vi "Stepper_motor_control_labview_version_2.0.vi"() -> ()   [LabVIEW 2019]
uses:
  <vilib>/Analysis/baseanly.llb/Mean (DBL).vi
  <vilib>/Waveform/WDTOps.llb/WDT Append Waveforms DBL.vi
  <vilib>/Analysis/NI_AALBase.lvlib
panel:
  out "Distance in cm":dbl
  in  "Stop Sensor CCW":bool
  out "Waveform Chart":waveform(dbl)(graph)
  in  "Stop sensor CW":bool
  in  "CW":bool
  out "DO CW":bool[](array[boolean])
  in  "How many laps CW":i32
  in  "How many laps CCW":i32
  in  "CCW":bool
  out "DO CCW":bool[](array[boolean])
  # "4 Steg = 1,8 x 4 = 7,2\n=> 45/7,2 = 6,25 = 25 varv\n=> 90/7,2 = 12.5 = 50 varv\n=> 360/7,2 = 50 = 200 varv"
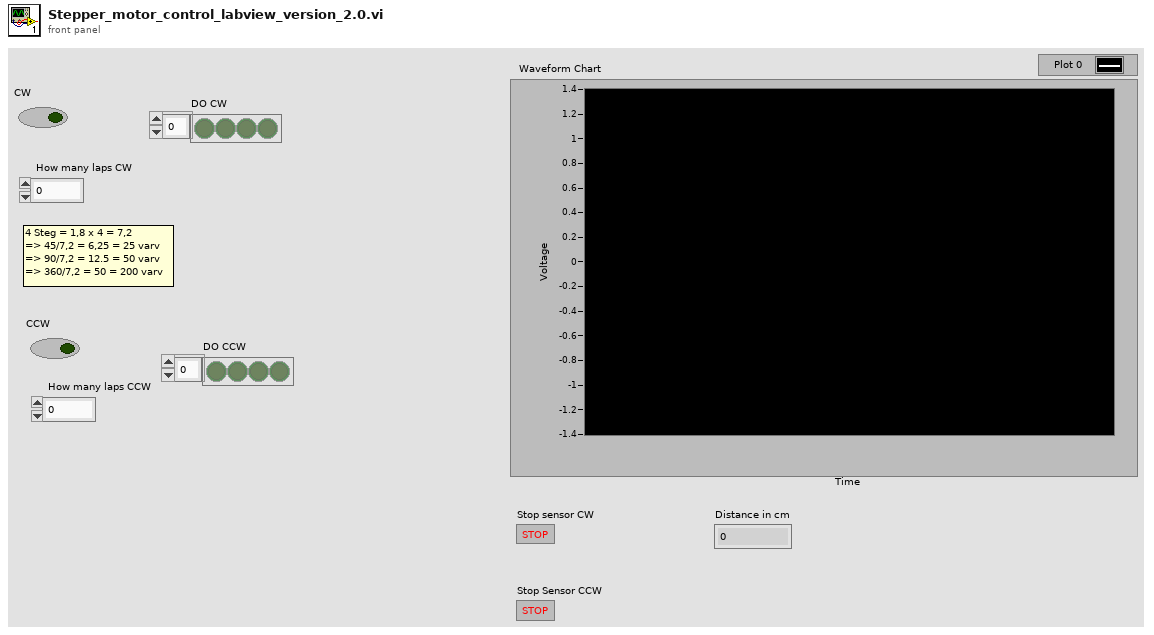
[diagram p1: front panel]
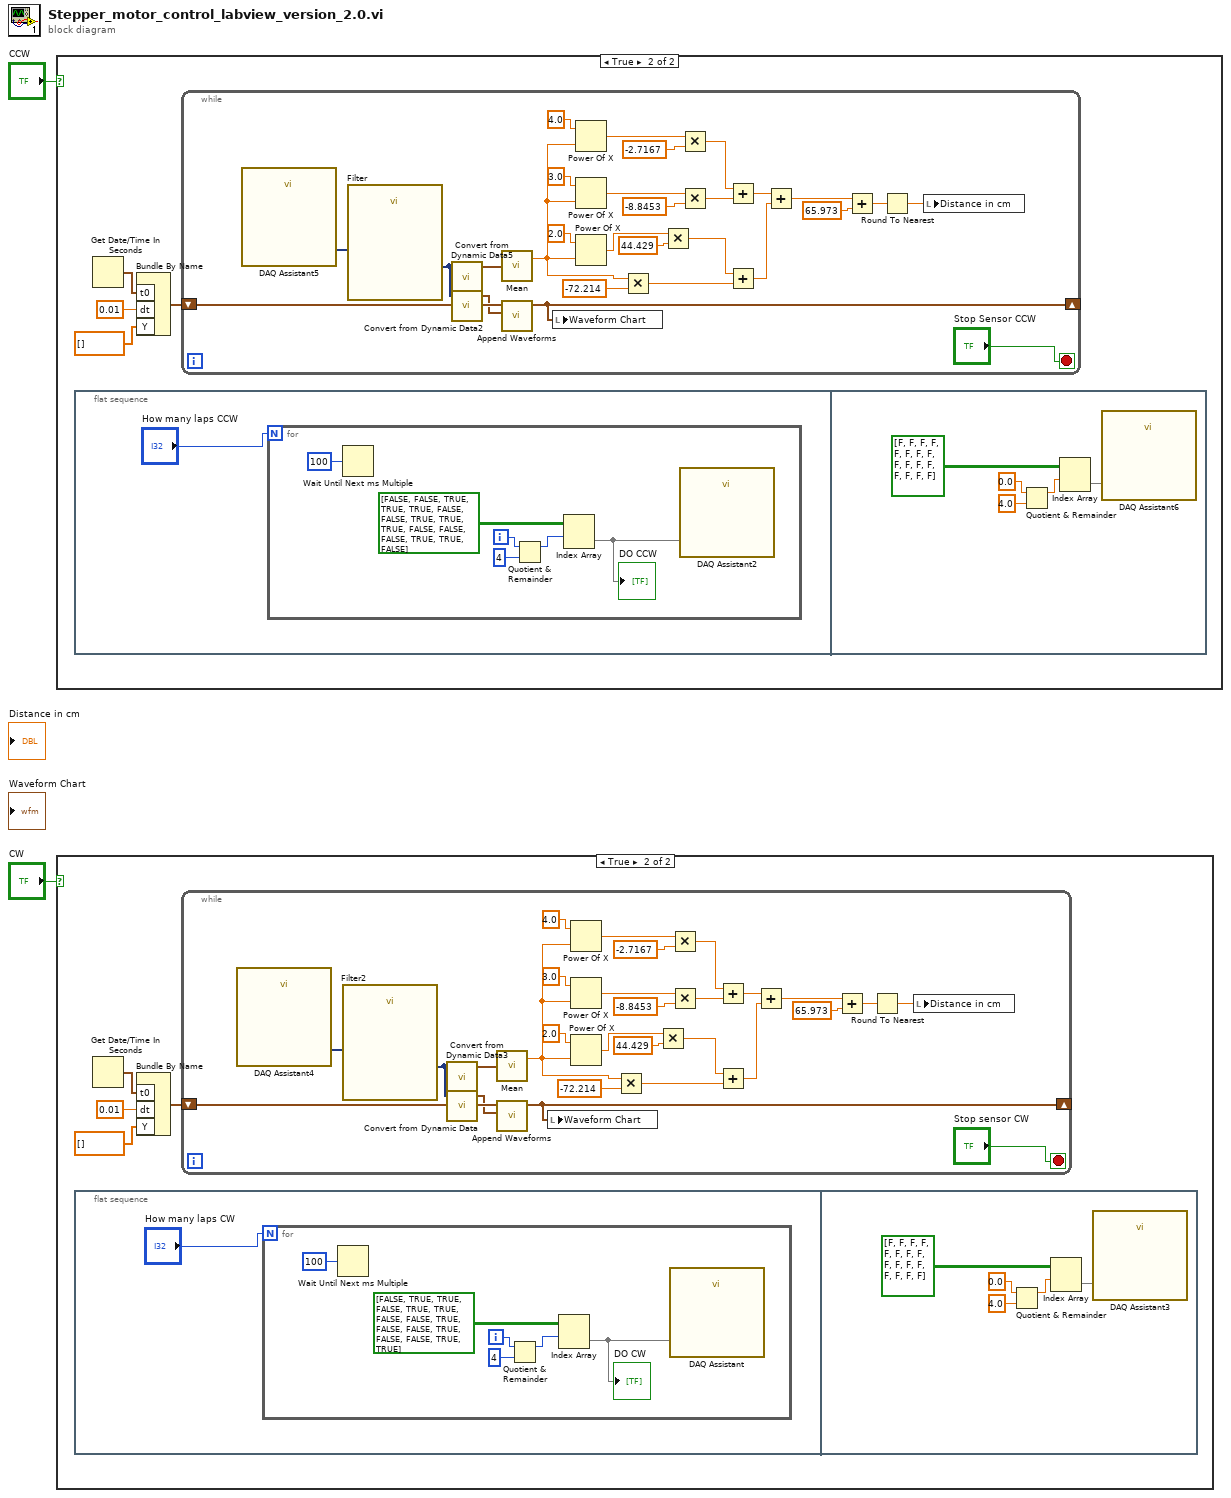
[diagram p0: block diagram]
diagram:
  n1 = case shown="True" "CCW" {
    frame False {
    }
    frame True {
      n2 = flat-sequence {
        frame #0 {
          n3 = for {
            N: "How many laps CCW" -> [_]
            i -> [w13]
            n4 = Wait Until Next ms Multiple(millisecond multiple=u32 100) -> ()  [unwired: 1 out]
            n5 = Quotient & Remainder(x=w13, y=4) -> (x-y*floor(x/y)=w11:i32)  [unwired: 1 out]
            n6 = Index Array(array=bool[][] [[FALSE, FALSE, TRUE, TRUE], [TRUE, FALSE, FALSE, TRUE], [TRUE, TRUE, FALSE, FALSE], [FALSE, TRUE, TRUE, FALSE]], index (row)=w11) -> (element=w10:bool[])  [unwired: 1 in]
            "DO CCW" <- w10
            n7 = call "DAQ Assistant2"("data"=w10) -> ()  [unwired: 17 in, 2 out]
          }
        }
        frame #1 {
          n8 = Quotient & Remainder(x=0.0, y=4.0 ("x-y*floor(x/y)")) -> (x-y*floor(x/y)=w18:dbl)  [unwired: 1 out]
          n9 = Index Array(array=bool[][] [[FALSE, FALSE, FALSE, FALSE], [FALSE, FALSE, FALSE, FALSE], [FALSE, FALSE, FALSE, FALSE], [FALSE, FALSE, FALSE, FALSE]], index (row)=w18) -> (element=w17:bool[])  [unwired: 1 in]
          n10 = call "DAQ Assistant6"("data"=w17) -> ()  [unwired: 17 in, 2 out]
        }
      }
      n11 = Get Date/Time In Seconds() -> (seconds since 1Jan1904=w6:timestamp)
      n12 = Bundle By Name("t0"=w6, "dt"=0.01, "Y"=dbl[] []) -> (w5:waveform(dbl))  [unwired: 1 in]
      n13 = while {
        shift-right: [w43] -> _
        shift-left: w5 -> [w45]
        stop <- "Stop Sensor CCW" stop-if-true
        n14 = call "DAQ Assistant5"() -> ("data"=w22:dynamicdata)  [unwired: 17 in, 2 out]
        n15 = call "Filter"("Signal"=w22) -> ("Filtered Signal"=w20:dynamicdata)  [unwired: 9 in, 1 out]
        n16 = call "Convert from Dynamic Data5"("Dynamic Data Type"=w20) -> ("Array of Waveform"=w19:waveform(dbl)[])  [unwired: 3 in]
        n17 = call "Convert from Dynamic Data2"("Dynamic Data Type"=w20) -> ("Waveform"=w44:waveform(dbl))  [unwired: 3 in]
        n18 = call-poly <vilib>:"Mean.vi"("X"=w19) -> ("mean"=w21:dbl)  [unwired: 1 out]
        n19 = call-poly <vilib>:"Append Waveforms.vi"("waveform B"=w44, "waveform A"=w45) -> ("waveform out"=w43:waveform(dbl))  [unwired: 8 in, 1 out]
        n20 = local write "Waveform Chart"(w43) -> ()
        n21 = Power Of X(1:w21, 2:4.0 ("x^y")) -> (0:w41:dbl)
        n22 = Power Of X(1:w21, 2:3.0 ("y")) -> (0:w37:dbl)
        n23 = Power Of X(1:w21, 2:2.0 ("x^y")) -> (0:w36:dbl)
        n24 = Multiply(x=w21, y=-72.214) -> (x*y=w29:dbl)
        n25 = Multiply(x=w36, y=44.429) -> (x*y=w30:dbl)
        n26 = Multiply(x=w41, y=-2.7167) -> (x*y=w32:dbl)
        n27 = Multiply(x=w37, y=-8.8453) -> (x*y=w31:dbl)
        n28 = Add(x=w32, y=w31) -> (x+y=w28:dbl)
        n29 = Add(x=w30, y=w29) -> (x+y=w27:dbl)
        n30 = Add(x=w28, y=w27) -> (x+y=w25:dbl)
        n31 = Add(x=w25, y=65.973) -> (x+y=w24:dbl)
        n32 = Round To Nearest(number=w24) -> (nearest integer value=w23:dbl)
        n33 = local write "Distance in cm"(w23) -> ()
      }
    }
  }
  n34 = case shown="True" "CW" {
    frame False {
    }
    frame True {
      n35 = flat-sequence {
        frame #0 {
          n36 = for {
            N: "How many laps CW" -> [_]
            i -> [w57]
            n37 = Wait Until Next ms Multiple(millisecond multiple=u32 100) -> ()  [unwired: 1 out]
            n38 = Quotient & Remainder(x=w57, y=4) -> (x-y*floor(x/y)=w55:i32)  [unwired: 1 out]
            n39 = Index Array(array=bool[][] [[FALSE, TRUE, TRUE, FALSE], [TRUE, TRUE, FALSE, FALSE], [TRUE, FALSE, FALSE, TRUE], [FALSE, FALSE, TRUE, TRUE]], index (row)=w55) -> (element=w54:bool[])  [unwired: 1 in]
            "DO CW" <- w54
            n40 = call "DAQ Assistant"("data"=w54) -> ()  [unwired: 17 in, 2 out]
          }
        }
        frame #1 {
          n41 = Quotient & Remainder(x=0.0, y=4.0 ("x-y*floor(x/y)")) -> (x-y*floor(x/y)=w61:dbl)  [unwired: 1 out]
          n42 = Index Array(array=bool[][] [[FALSE, FALSE, FALSE, FALSE], [FALSE, FALSE, FALSE, FALSE], [FALSE, FALSE, FALSE, FALSE], [FALSE, FALSE, FALSE, FALSE]], index (row)=w61) -> (element=w62:bool[])  [unwired: 1 in]
          n43 = call "DAQ Assistant3"("data"=w62) -> ()  [unwired: 17 in, 2 out]
        }
      }
      n44 = Get Date/Time In Seconds() -> (seconds since 1Jan1904=w49:timestamp)
      n45 = Bundle By Name("t0"=w49, "dt"=0.01, "Y"=dbl[] []) -> (w50:waveform(dbl))  [unwired: 1 in]
      n46 = while {
        shift-right: [w87] -> _
        shift-left: w50 -> [w89]
        stop <- "Stop sensor CW" stop-if-true
        n47 = call "DAQ Assistant4"() -> ("data"=w66:dynamicdata)  [unwired: 17 in, 2 out]
        n48 = call "Filter2"("Signal"=w66) -> ("Filtered Signal"=w65:dynamicdata)  [unwired: 9 in, 1 out]
        n49 = call "Convert from Dynamic Data3"("Dynamic Data Type"=w65) -> ("Array of Waveform"=w64:waveform(dbl)[])  [unwired: 3 in]
        n50 = call "Convert from Dynamic Data"("Dynamic Data Type"=w65) -> ("Waveform"=w88:waveform(dbl))  [unwired: 3 in]
        n51 = call-poly <vilib>:"Mean.vi"("X"=w64) -> ("mean"=w63:dbl)  [unwired: 1 out]
        n52 = call-poly <vilib>:"Append Waveforms.vi"("waveform B"=w88, "waveform A"=w89) -> ("waveform out"=w87:waveform(dbl))  [unwired: 8 in, 1 out]
        n53 = local write "Waveform Chart"(w87) -> ()
        n54 = Power Of X(1:w63, 2:4.0 ("x^y")) -> (0:w77:dbl)
        n55 = Power Of X(1:w63, 2:3.0 ("y")) -> (0:w78:dbl)
        n56 = Power Of X(1:w63, 2:2.0 ("x^y")) -> (0:w79:dbl)
        n57 = Multiply(x=w63, y=-72.214) -> (x*y=w83:dbl)
        n58 = Multiply(x=w79, y=44.429) -> (x*y=w82:dbl)
        n59 = Multiply(x=w77, y=-2.7167) -> (x*y=w80:dbl)
        n60 = Multiply(x=w78, y=-8.8453) -> (x*y=w81:dbl)
        n61 = Add(x=w80, y=w81) -> (x+y=w84:dbl)
        n62 = Add(x=w82, y=w83) -> (x+y=w85:dbl)
        n63 = Add(x=w84, y=w85) -> (x+y=w86:dbl)
        n64 = Add(x=w86, y=65.973) -> (x+y=w68:dbl)
        n65 = Round To Nearest(number=w68) -> (nearest integer value=w67:dbl)
        n66 = local write "Distance in cm"(w67) -> ()
      }
    }
  }
